vi "Main.vi"() -> ()   [LabVIEW 2013]
uses:
  <vilib>/Utility/error.llb/DialogType.ctl
panel:
  in  "IP-Адрес блока синхронизации":string="172.16.21.75"
  out "Синхроимпульс":bool
  out "conn sync":refnum<k5>
  out "conn src":refnum<k5>
  in  "Ручное управление":bool=TRUE
  in  "мс":u16=2000 min=100 max=60000 step=100
  in  "stop":bool
  out "message":string=" INSTRUCTIONS:\r\rNormal Use:  When using subVIs that incorporate the error in/error out (or error I/O) structure, place this handler where you want to inform the user of an error, typically at the end of the I/O data path, as the last action of the program.  If the error in error? is ERROR, the handler creates a message describing the error and its source.  If the type of dialog = 1 (default), the message is displayed to the user, who can only acknowedge it.  If the type = 2, the user can acknowledge the message or abort execution; aborting a program with active I/O is not recommended.  If the type = 0, no message is displayed; this is used to process the error programmatically, and the error out cluster elements are wired to individual terminals for that reason.  \r\rOther Use:\n\r\nlocal testing.  To test the error code of a subVI or function that does not have the error I/O structure, you can wire its error code and a source string to the local error code and error source inputs.  If error in error? indicates no error and error code is not equal to 0, the local code and source are substituted for the error in values, and error? is set TRUE (ERROR)."
  in  "В":dbl step=1.0 format="%.3f"
  in  "А":dbl step=1.0 format="%.3f"
  in  "NeedToSetVoltage":bool
  in  "NeedToSetCurrent":bool
  out "U вых,В":string
  out "I вых,А":string
  in  "Ручное вкл.":bool
  out "Выход":bool
  in  "IP-Адрес источника":string="172.16.21.205"
  # "Управление питанием корректора на выходе RFQ"
  # "Уставка"
  # "Длительность \n   импульса при \nавтоматич. управлении"
  # "Выход источника"
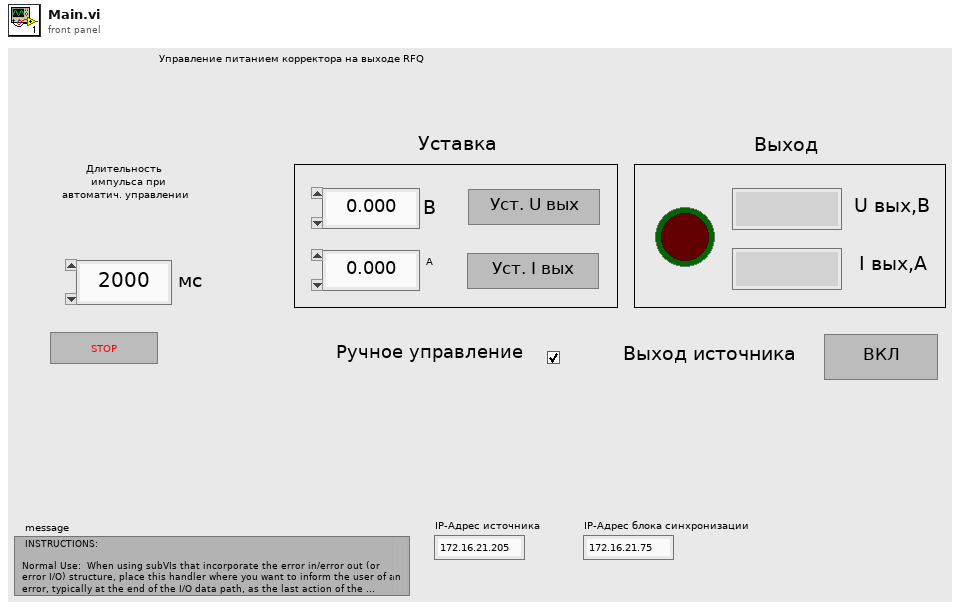
[diagram p1: front panel]
types:
  T1 = typedef "DialogType.ctl" = u16
  T2 = enum16{"Standard", "Buffered", "CRLF", "Immediate"}
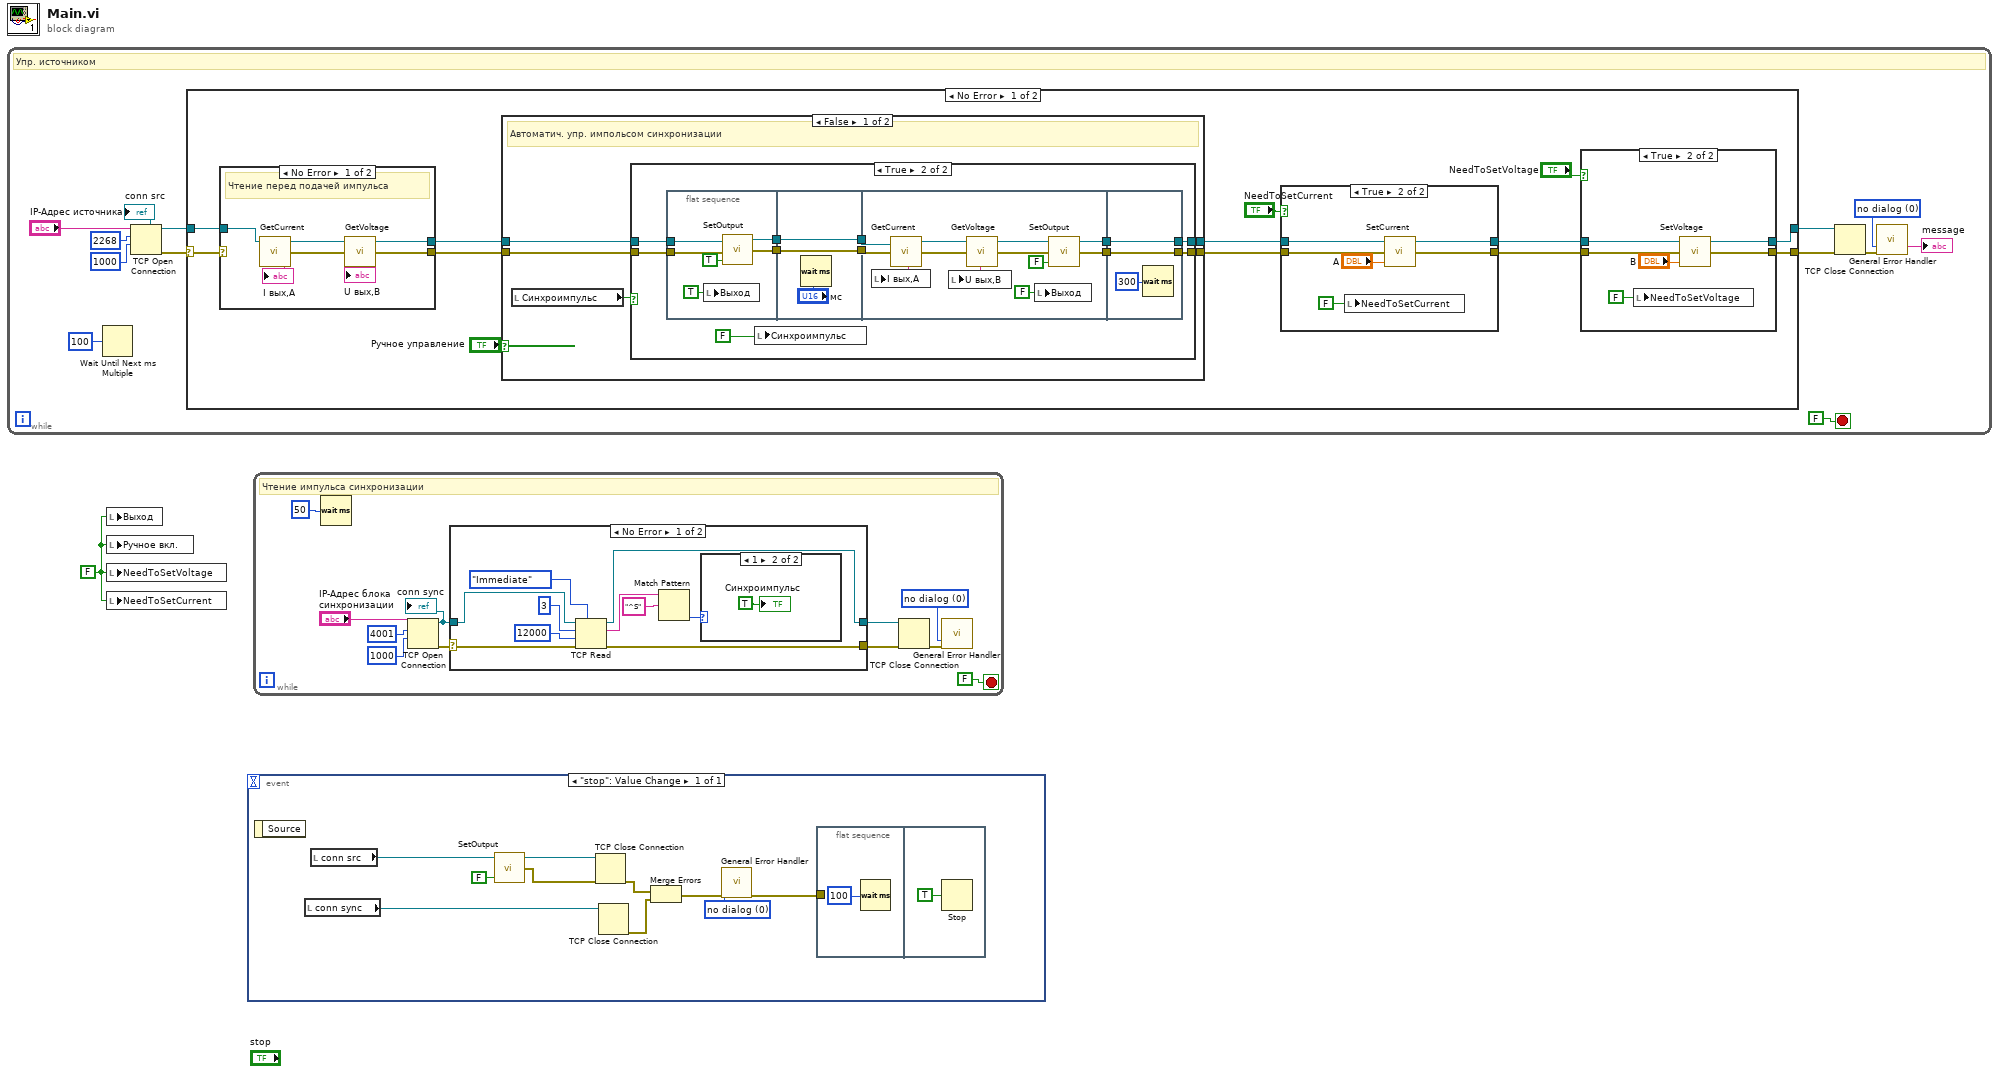
[diagram p0: block diagram]
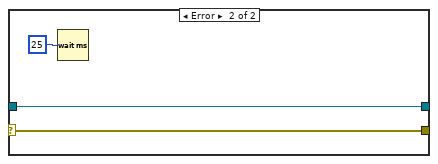
[diagram p3: hidden frame]
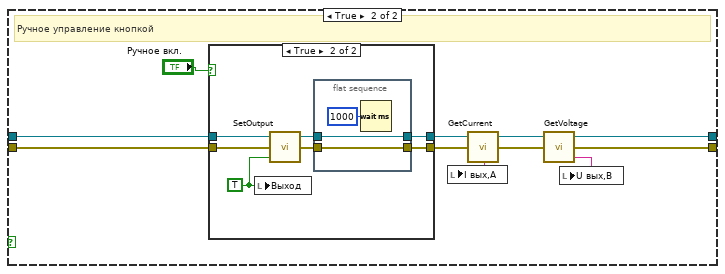
[diagram p5: hidden frame]
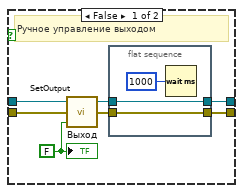
[diagram p6: hidden frame]
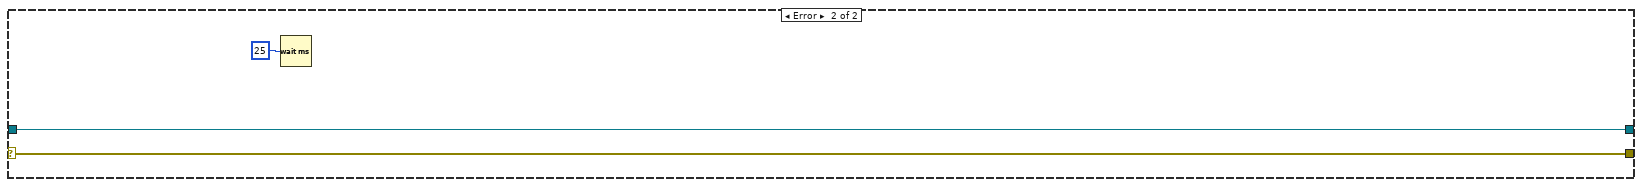
[diagram p10: hidden frame]
diagram:
  w1 = FALSE ("Connect")
  n1 = while {
    stop <- FALSE stop-if-true
    w5 = T1 0 items=["no dialog", "OK message", "continue or stop message", "OK message + warnings", "continue/stop + warnings"] ("type of dialog (OK msg:1)")
    # "Упр. источником"
    n2 = Wait Until Next ms Multiple(millisecond multiple=u32 100 ("milliseconds to wait")) -> ()  [unwired: 1 out]
    n3 = TCP Open Connection(address="IP-Адрес источника", remote port or service name=u16 2268 ("Port"), timeout ms (60000)=1000) -> (connection ID=w9:refnum<k5>, error out=w10:errorcluster)  [unwired: 1 in, 1 out]
    "conn src" <- w9
    n4 = case shown="No Error" w10 {
      selector: w10 -> [w20 w125]
      tunnel: w9 -> [w19 w126]
      tunnel: [w22 w126] -> w8
      tunnel: [w21 w125] -> w7
      frame No Error {
        n5 = case shown="No Error" w20 {
          selector: w20 -> [_ w107]
          tunnel: w19 -> [w102 w108]
          tunnel: [w101 w107] -> w18
          tunnel: [w100 w108] -> w17
          frame No Error {
            # "Чтение перед подачей импульса"
            n6 = call "GetCurrent.vi"("connection ID"=w102) -> ("Current"=→"I вых,А":string, "error out"=w103:errorcluster, "connection ID out"=w105:refnum<k5>)  [unwired: 1 in, 1 out]
            n7 = call "GetVoltage.vi"("error in"=w103, "connection ID"=w105) -> ("Voltage"=→"U вых,В":string, "error out"=w101:errorcluster, "connection ID out"=w100:refnum<k5>)  [unwired: 1 out]
          }
          frame Error {
          }
        }
        n8 = case shown="False" "Ручное управление" {
          tunnel: w18 -> [w30 w79]
          tunnel: w17 -> [w31 w78]
          tunnel: [w29 w71] -> w15
          tunnel: [w28 w70] -> w14
          frame False {
            # "Автоматич. упр. импольсом синхронизации"
            n9 = local read "Синхроимпульс"() -> (w27:bool)
            n10 = case shown="True" w27 {
              tunnel: w31 -> [w33 w44]
              tunnel: w30 -> [w32 w43]
              tunnel: [w33 w38] -> w29
              tunnel: [w32 w37] -> w28
              frame False {
              }
              frame True {
                n11 = flat-sequence {
                  tunnel: w44 -> [w49]
                  tunnel: w43 -> [w48]
                  tunnel: [w46] -> w41
                  tunnel: [w45] -> w39
                  tunnel: [w52] -> w42
                  tunnel: w41 -> [w52]
                  tunnel: [w51] -> w40
                  tunnel: w39 -> [w51]
                  tunnel: w42 -> [w58]
                  tunnel: w40 -> [w57]
                  tunnel: [w63] -> w36
                  tunnel: [w62] -> w35
                  tunnel: [w67] -> w37
                  tunnel: [w68] -> w38
                  tunnel: w36 -> [w68]
                  tunnel: w35 -> [w67]
                  frame #0 {
                    n12 = local write "Выход"(TRUE ("ВКЛ ручное")) -> ()
                    n13 = call "SetOutput.vi"("State"=TRUE, "error in"=w48, "connection ID"=w49) -> ("error out"=w45:errorcluster, "connection ID out"=w46:refnum<k5>)  [unwired: 1 out]
                  }
                  frame #1 {
                    n14 = Wait (ms)(milliseconds to wait="мс") -> ()  [unwired: 1 out]
                  }
                  frame #2 {
                    n15 = call "GetCurrent.vi"("error in"=w57, "connection ID"=w58) -> ("Current"=w61:string, "error out"=w59:errorcluster, "connection ID out"=w60:refnum<k5>)  [unwired: 1 out]
                    n16 = local write "I вых,А"(w61) -> ()
                    n17 = call "GetVoltage.vi"("error in"=w59, "connection ID"=w60) -> ("Voltage"=w54:string, "error out"=w55:errorcluster, "connection ID out"=w56:refnum<k5>)  [unwired: 1 out]
                    n18 = local write "U вых,В"(w54) -> ()
                    n19 = local write "Выход"(FALSE ("ВКЛ ручное")) -> ()
                    n20 = call "SetOutput.vi"("State"=FALSE, "error in"=w55, "connection ID"=w56) -> ("error out"=w62:errorcluster, "connection ID out"=w63:refnum<k5>)  [unwired: 1 out]
                  }
                  frame #3 {
                    n21 = Wait (ms)(milliseconds to wait=u32 300) -> ()  [unwired: 1 out]
                  }
                }
                n22 = local write "Синхроимпульс"(FALSE ("NeedToSetOutput")) -> ()
              }
            }
          }
          frame True {
            # "Ручное управление кнопкой"
            n23 = case shown="True" "Ручное вкл." {
              tunnel: w79 -> [w84 w96]
              tunnel: w78 -> [w83 w95]
              tunnel: [w82 w93] -> w75
              tunnel: [w81 w91] -> w74
              frame False {
                w80 = FALSE ("State")
                # "Ручное управление выходом"
                n24 = call "SetOutput.vi"("State"=w80, "error in"=w84, "connection ID"=w83) -> ("error out"=w85:errorcluster, "connection ID out"=w86:refnum<k5>)  [unwired: 1 out]
                n25 = flat-sequence {
                  tunnel: w86 -> [w89]
                  tunnel: [w89] -> w82
                  tunnel: w85 -> [w88]
                  tunnel: [w88] -> w81
                  frame #0 {
                    n26 = Wait (ms)(milliseconds to wait=u32 1000) -> ()  [unwired: 1 out]
                  }
                }
                "Выход" <- w80
              }
              frame True {
                w90 = TRUE ("State")
                n27 = local write "Выход"(w90) -> ()
                n28 = call "SetOutput.vi"("State"=w90, "error in"=w96, "connection ID"=w95) -> ("error out"=w92:errorcluster, "connection ID out"=w94:refnum<k5>)  [unwired: 1 out]
                n29 = flat-sequence {
                  tunnel: w94 -> [w99]
                  tunnel: [w99] -> w93
                  tunnel: w92 -> [w98]
                  tunnel: [w98] -> w91
                  frame #0 {
                    n30 = Wait (ms)(milliseconds to wait=u32 1000) -> ()  [unwired: 1 out]
                  }
                }
              }
            }
            n31 = call "GetCurrent.vi"("error in"=w74, "connection ID"=w75) -> ("Current"=w76:string, "error out"=w72:errorcluster, "connection ID out"=w73:refnum<k5>)  [unwired: 1 out]
            n32 = local write "I вых,А"(w76) -> ()
            n33 = call "GetVoltage.vi"("error in"=w72, "connection ID"=w73) -> ("Voltage"=w69:string, "error out"=w70:errorcluster, "connection ID out"=w71:refnum<k5>)  [unwired: 1 out]
            n34 = local write "U вых,В"(w69) -> ()
          }
        }
        n35 = case shown="True" "NeedToSetCurrent" {
          tunnel: [w118 w123] -> w26
          tunnel: [w117 w121] -> w23
          tunnel: w15 -> [w118 w120]
          tunnel: w14 -> [w117 w119]
          frame False {
          }
          frame True {
            n36 = local write "NeedToSetCurrent"(FALSE ("NeedToSetOutput")) -> ()
            n37 = call "SetCurrent.vi"("Current"="А", "error in"=w119, "connection ID"=w120) -> ("error out"=w121:errorcluster, "connection ID out"=w123:refnum<k5>)  [unwired: 1 out]
          }
        }
        n38 = case shown="True" "NeedToSetVoltage" {
          tunnel: w26 -> [w110 w116]
          tunnel: [w110 w113] -> w22
          tunnel: w23 -> [w109 w112]
          tunnel: [w109 w111] -> w21
          frame False {
          }
          frame True {
            n39 = local write "NeedToSetVoltage"(FALSE ("NeedToSetOutput")) -> ()
            n40 = call "SetVoltage.vi"("Voltage"="В", "error in"=w112, "connection ID"=w116) -> ("error out"=w111:errorcluster, "connection ID out"=w113:refnum<k5>)  [unwired: 1 out]
          }
        }
      }
      frame Error {
        n41 = Wait (ms)(milliseconds to wait=u32 25) -> ()  [unwired: 1 out]
      }
    }
    n42 = TCP Close Connection(connection ID=w8, error in (no error)=w7) -> (error out=w6:errorcluster)  [unwired: 2 out]
    n43 = call <vilib>:"General Error Handler.vi"("type of dialog (OK msg:1)"=w5, "error in (no error)"=w6) -> ("message"=→"message":string)  [unwired: 9 in, 4 out]
  }
  n44 = local write "Выход"(w1) -> ()
  n45 = local write "Ручное вкл."(w1) -> ()
  n46 = local write "NeedToSetVoltage"(w1) -> ()
  n47 = local write "NeedToSetCurrent"(w1) -> ()
  n48 = event shown="[0] \"stop\": Value Change" {
    selector: _ -> [_]
    dyn-events: _ -> [_]
    timeout: _ -> [_]
    event "stop": Value Change {
      w133 = T1 0 items=["no dialog", "OK message", "continue or stop message", "OK message + warnings", "continue/stop + warnings"] ("type of dialog (OK msg:1)")
      n49 = event-data() -> ()  [unwired: 1 in, 1 out]
      n50 = local read "conn sync"() -> (w137:refnum<k5>)
      n51 = local read "conn src"() -> (w131:refnum<k5>)
      n52 = call "SetOutput.vi"("State"=FALSE, "connection ID"=w131) -> ("error out"=w129:errorcluster, "connection ID out"=w130:refnum<k5>)  [unwired: 1 in, 1 out]
      n53 = TCP Close Connection(connection ID=w130, error in (no error)=w129) -> (error out=w136:errorcluster)  [unwired: 1 in, 1 out]
      n54 = TCP Close Connection(connection ID=w137) -> (error out=w135:errorcluster)  [unwired: 2 in, 1 out]
      n55 = Merge Errors(w136, w135) -> (w134:errorcluster)
      n56 = call <vilib>:"General Error Handler.vi"("type of dialog (OK msg:1)"=w133, "error in (no error)"=w134) -> ("error out"=w132:errorcluster)  [unwired: 9 in, 4 out]
      n57 = flat-sequence {
        tunnel: w132 -> [_]
        frame #0 {
          n58 = Wait (ms)(milliseconds to wait=u32 100) -> ()  [unwired: 1 out]
        }
        frame #1 {
          n59 = Stop(stop? (T)=TRUE) -> ()
        }
      }
    }
  }
  n60 = while {
    stop <- FALSE stop-if-true
    w143 = T1 0 items=["no dialog", "OK message", "continue or stop message", "OK message + warnings", "continue/stop + warnings"] ("type of dialog (OK msg:1)")
    # "Чтение импульса синхронизации"
    n61 = Wait (ms)(milliseconds to wait=u32 50) -> ()  [unwired: 1 out]
    n62 = TCP Open Connection(address="IP-Адрес блока синхронизации", remote port or service name=u16 4001 ("Port"), timeout ms (60000)=1000) -> (connection ID=w141:refnum<k5>, error out=w147:errorcluster)  [unwired: 1 in, 1 out]
    "conn sync" <- w141
    n63 = case shown="No Error" w147 {
      selector: w147 -> [w158 w162]
      tunnel: w141 -> [w160 w163]
      tunnel: [w155 w163] -> w146
      tunnel: [w156 w162] -> w145
      frame No Error {
        n64 = TCP Read(connection ID=w160, bytes to read=3, error in (no error)=w158, 7:T2."Immediate" ("mode (standard)"), 9:12000 ("timeout ms (25000)")) -> (connection ID out=w155:refnum<k5>, data out=w153:string, error out=w156:errorcluster)
        n65 = Match Pattern(string=w153, regular expression="^S") -> (offset past match=w151:i32)  [unwired: 1 in, 3 out]
        n66 = case shown="1" w151 {
          frame -1, Default {
          }
          frame 1 {
            "Синхроимпульс" <- TRUE ("NeedToSetOutput")
          }
        }
      }
      frame Error {
        n67 = Wait (ms)(milliseconds to wait=u32 25) -> ()  [unwired: 1 out]
      }
    }
    n68 = TCP Close Connection(connection ID=w146, error in (no error)=w145) -> (error out=w144:errorcluster)  [unwired: 2 out]
    n69 = call <vilib>:"General Error Handler.vi"("type of dialog (OK msg:1)"=w143, "error in (no error)"=w144) -> ()  [unwired: 9 in, 5 out]
  }
